vi "Global_Joystick Manipulator.vi"() -> ()   [LabVIEW 2017, in "Joystick.lvlib"]
uses:
  Joystick.lvlib
panel:
  out "Joystick_SEN_POVs_Man":i16[](array[numeric])
  out "Joystick_SEN_Buttons_Man":bool[](array[boolean])
  out "Joystick_SEN_Axes_Man":dbl[](array[numeric])
  # "The Names of the Data items in the Global Variable MUST describe who the Single Writer is\nNaming Convention of all Data Items is:   Lib Name_Loop Name (SM or SEN or ACT)_Data Name\nExample   Drive_ACT_X axis;  GameController_SEN_JoystickLeft;  Hopper_SM_AgitatorSpeed"
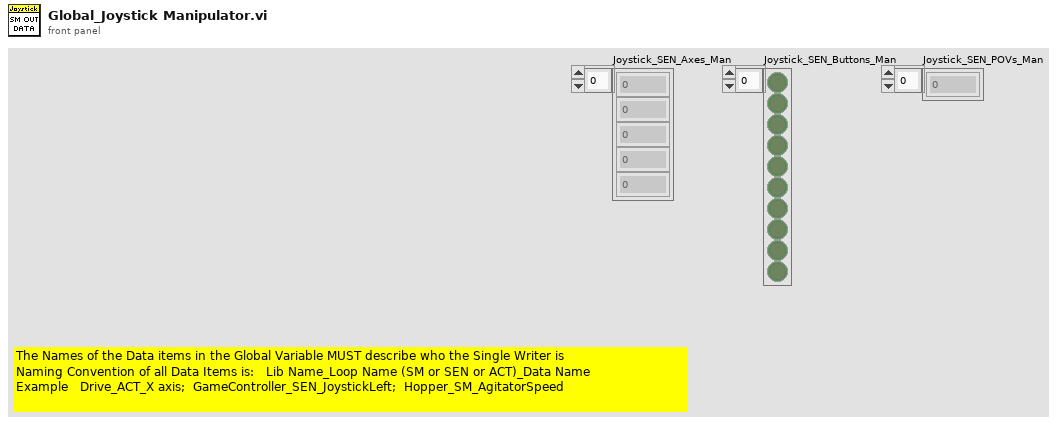
[diagram p1: front panel]
diagram:
